vi "Add Documentation to Initialize VI.vi"   [LabVIEW 2015]
doc: "<b> </b> <b> </b>\n©2016 Q Software Innovations, LLC (QSI)\nwritten by Quentin Alldredge\nproduced in LabVIEW 2015"
uses:
  Project Manipulation Scripts/Project Manipulation Scripts.lvlib
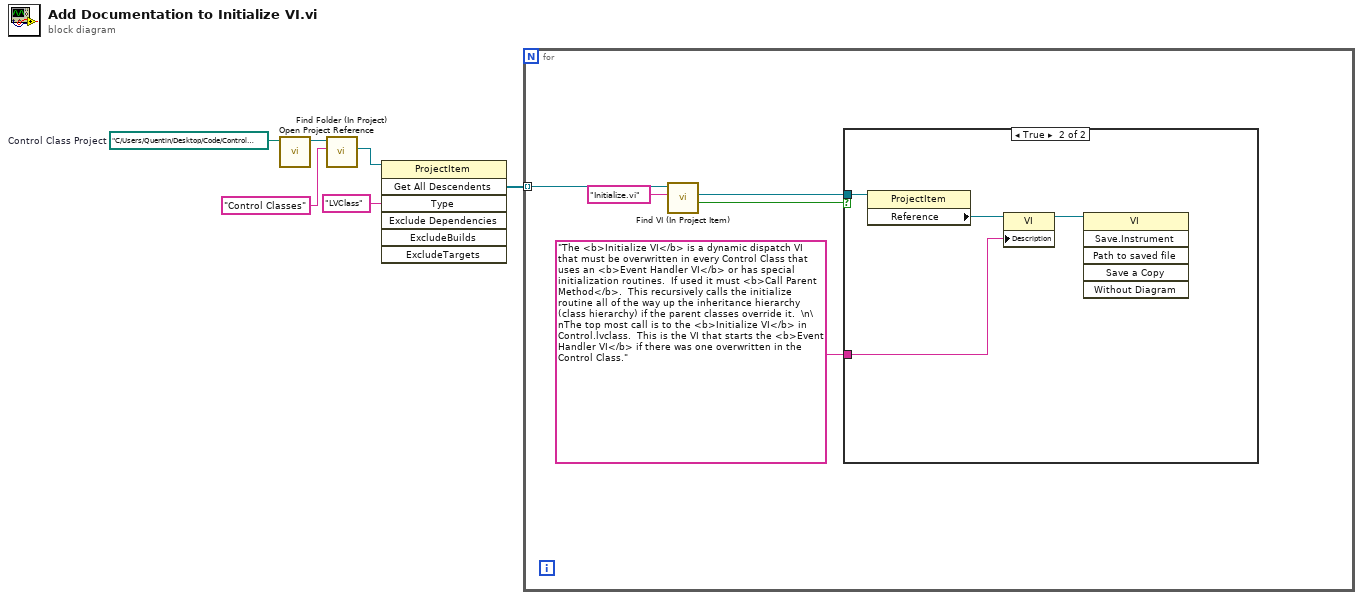
[diagram p0: block diagram]
diagram:
  w6 = path "C:/Users/Quentin/Desktop/Code/Control Class Toolkit/Control Class Toolkit.lvproj"  # Control Class Project
  n1 = call "Open Project Reference.vi"("Project Path"=w6) -> ("Project out"=w5:refnum<vi>)  [unwired: 10 in]
  n2 = call "Find Folder (In Project).vi"("Folder Name"="Control Classes", "Project in"=w5) -> ("Folder Refnum"=w3:refnum<vi>)  [unwired: 7 in, 2 out]
  n3 = invoke class="ProjectItem" method="Get All Descendents"(reference=w3, "Type"="LVClass") -> ("All Descendents"=w1:refnum<vi>[])  [unwired: 5 in, 6 out]
  n4 = for {
    tunnel: w1 -> [w11] mode=indexing
    n5 = call "Find VI (In Project Item).vi"("VI Name"="Initialize.vi", "ProjectItem in"=w11) -> ("Found?"=w7:bool, "VI ProjectItem Refnum"=w9:refnum<vi>)  [unwired: 7 in, 1 out]
    n6 = case shown="True" w7 {
      tunnel: w9 -> [_ w15]
      tunnel: "The <b>Initialize VI</b> is a dynamic dispatch VI that must be overwritten in every Control Class that uses an <b>Event Handler VI</b> or has special initialization routines.  If used it must <b>Call Parent Method</b>.  This recursively calls the initialize routine all of the way up the inheritance hierarchy (class hierarchy) if the parent classes override it.  \n\nThe top most call is to the <b>Initialize VI</b> in Control.lvclass.  This is the VI that starts the <b>Event Handler VI</b> if there was one overwritten in the Control Class." ("VI Description") -> [_ w13]
      frame False {
      }
      frame True {
        n7 = property class="ProjectItem"(reference=w15) -> ("Reference"=w14:refnum<vi>)  [unwired: 1 in, 2 out]
        n8 = property class="VI"(reference=w14, "Description"=w13) -> (reference out=w12:refnum<vi>)  [unwired: 1 in, 1 out]
        n9 = invoke class="VI" method="Save.Instrument"(reference=w12) -> ()  [unwired: 5 in, 6 out]
      }
    }
  }
